vi "Input Queue Ref Holder.vi"(7 "Hold":bool, 8 "error in (no error)":errorcluster, 11 "Message Queue In":refnum<queue>) -> (0 "error out":errorcluster, 3 "Input Message Queue":refnum<queue>)   [LabVIEW 2015, in "PL Model.lvlib"]
uses:
  PL Model.lvlib
  support/Message Queue/Message Cluster.ctl
  support/Message Queue/PLC Message Queue.lvlib
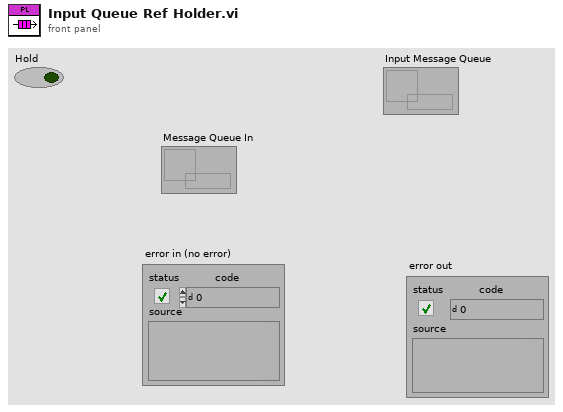
[diagram p1: front panel]
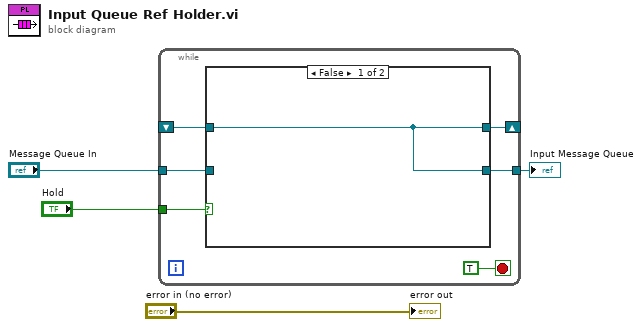
[diagram p0: block diagram]
diagram:
  n1 = while {
    shift-right: [w8] -> _
    shift-left: _ -> [w5]
    tunnel: "Message Queue In" -> [w7]
    tunnel: "Hold" -> [w9]
    tunnel: [w6] -> w2
    stop <- TRUE stop-if-true
    n2 = case shown="False" w9 {
      tunnel: [w11 w12] -> w8
      tunnel: w7 -> [_ w12]
      tunnel: [w11 w12] -> w6
      tunnel: w5 -> [w11 _]
      frame False {
      }
      frame True {
      }
    }
  }
  "Input Message Queue" <- w2
  "error out" <- "error in (no error)"
